vi "subFD_StructSel & CoefQuant.vi"() -> ()   [LabVIEW 2023]
uses:
  <vilib>/addons/Digital Filter Design/_Objects.llb/DFD Pole-Zero Plot.ctl
  <vilib>/addons/Digital Filter Design/_Objects.llb/DFD Filter Obj.ctl
  <vilib>/addons/Digital Filter Design/_Objects.llb/DFD Filter Coef.ctl
  <vilib>/addons/Digital Filter Design/_Objects.llb/DFD Filter Structure Type Selector.ctl
  <vilib>/addons/Digital Filter Design/_Objects.llb/dfd_Internal Quantization Settings.ctl
  <vilib>/addons/Digital Filter Design/_Objects.llb/dfd_Internal Quantization Srcs.ctl
  <vilib>/addons/Digital Filter Design/_Objects.llb/DFD Coef Norm Type.ctl
  <vilib>/addons/Digital Filter Design/_Objects.llb/DFD Phase Setting.ctl
  <vilib>/addons/Digital Filter Design/FXPModel.llb/DFD FXP Get Quantizer (All).vi
  <vilib>/addons/Digital Filter Design/FXPModel.llb/DFD FXP Quantize Coef (Easy).vi
  <vilib>/addons/Digital Filter Design/Analysis.llb/DFD Plot Freq Response (Linear-Spaced).vi
  <vilib>/addons/Digital Filter Design/NI_DigFilterLicensed.lvlib
panel:
  in  "Scale Type":u16(ring) items=["No Norm", "Time Domain 1-Norm", "Time Domain 2-Norm", "Time Domain Inf-Norm"]
  out "Status":string="Calculating........"
  in  "Scale Filter before Quantization":bool=TRUE
  in  "Coefficients a/k Word Length":i16=16 min=1 max=32 step=1
  in  "Coefficients b/v Word Length":i16=16 min=1 max=32 step=1
  out "Coefficients Report":string
  in  "Target Structure":u16(ring)=1 items=["FIR Direct Form"=1, "FIR Direct Form Transposed"=2, "FIR Symmetric"=3, "FIR Antisymmetric"=4, "IIR Direct Form I"=5, "IIR Direct Form I Transposed"=6, "IIR Direct Form II"=7, "IIR Direct Form II Transposed"=8, "IIR Cascaded Second-Order Sections Form I"=9, "IIR Cascaded Second-Order Sections Form I Transposed"=10, "IIR Cascaded Second-Order Sections Form II"=11, "IIR Cascaded Second-Order Sections Form II Transposed"=12, "Lattice Allpass (basic sections)"=13, "Lattice Allpass (one multiplier sections)"=14, "Lattice Allpass (normalized sections)"=15, "Lattice AR (basic sections)"=16, "Lattice AR (one multiplier sections)"=17, "Lattice AR (normalized sections)"=18, "Lattice MA (minimum phase)"=19, "Lattice MA (maximum phase)"=20, "Lattice ARMA (basic sections)"=21, "Lattice ARMA (one multiplier sections)"=22, "Lattice ARMA (normalized sections)"=23]
  out "Successful Design?":bool
  out "filter out":T1={"mSRate_Fs"=1.0, "mSRate_Version"="1.0", "mSRate_Comments"="", "mSRate_OrgCoef"={"type"=enum."Undefined", "gain"=1.0, "coef a (k)"=[], "coef b (v)"=[]}, "mSRate_CurCoef"={"type"=enum."Undefined", "gain"=1.0, "coef a (k)"=[], "coef b (v)"=[]}, "mSRate_Quantized?"=FALSE, "mSRate_QCoef"={"type"=enum."Undefined", "gain"=1.0, "coef a (k)"=[], "coef b (v)"=[]}, "mSRate_QSettings"=[], "mSRate_Order"=0, "mSRate_Scaling"={"mSRate_ScaleByPowerOf2?"=FALSE, "mSRate_ScaleType"=enum."No Norm"}} {"mSRate_QSettings"."source" items=["Coef a/k"=0, "Coef b/v"=7, "Input"=1, "Output"=2, "Multiplicand"=3, "Product"=4, "Sum"=5, "Delay"=6, "Gain"=8]}
  in  "filter in":T1={"mSRate_Fs"=1.0, "mSRate_Version"="1.0", "mSRate_Comments"="", "mSRate_OrgCoef"={"type"=enum."Undefined", "gain"=1.0, "coef a (k)"=[], "coef b (v)"=[]}, "mSRate_CurCoef"={"type"=enum."Undefined", "gain"=1.0, "coef a (k)"=[], "coef b (v)"=[]}, "mSRate_Quantized?"=FALSE, "mSRate_QCoef"={"type"=enum."Undefined", "gain"=1.0, "coef a (k)"=[], "coef b (v)"=[]}, "mSRate_QSettings"=[], "mSRate_Order"=0, "mSRate_Scaling"={"mSRate_ScaleByPowerOf2?"=FALSE, "mSRate_ScaleType"=enum."No Norm"}} {"mSRate_QSettings"."source" items=["Coef a/k"=0, "Coef b/v"=7, "Input"=1, "Output"=2, "Multiplicand"=3, "Product"=4, "Sum"=5, "Delay"=6, "Gain"=8]}
  in  "Graph Selector":u16(ring) items=["Magnitude", "Phase", "Group Delay", "Pole-Zero Plot", "Impulse Response"]
  in  "Unwrap?":bool=TRUE
  in  "Magnitude in dB?":bool=TRUE
  out "OK":bool
  in  "stop":bool
  out "Graph Tab":T7(tab)
  out "Magnitude Response":cluster{"f0":dbl, "df":dbl, "values":dbl[]}[](graph)
  out "Phase Response":cluster{"f0":dbl, "df":dbl, "values":dbl[]}[](graph)
  out "Group Delay":cluster{"f0":dbl, "df":dbl, "values":dbl[]}[](graph)
  out "Z-Plane":T8
  out "Coefficients":dbl[][](graph)
  # "Design Result"
  # "Target Structure"
  # "Coefficients Quantization Settings"
  # "Coefficients Report"
  # "Coefficients a/k\nWord Length"
  # "Coefficients b/v\nWord Length"
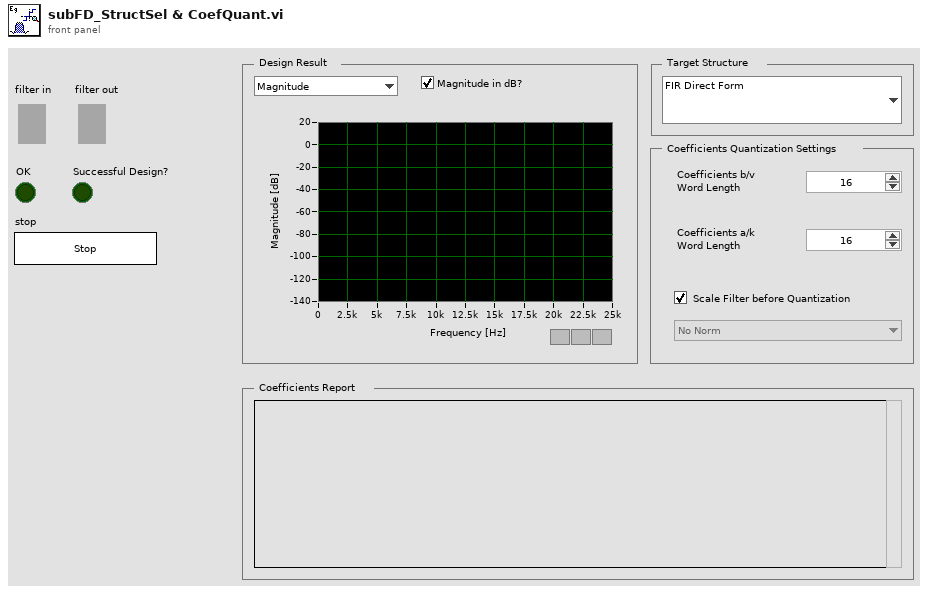
[diagram p1: front panel]
types:
  T1 = typedef "NI_DigFilterLicensed.lvlib/DFD Filter Obj.ctl" = cluster{"mSRate_Fs":dbl, "mSRate_Version":string, "mSRate_Comments":string, "mSRate_OrgCoef":T2, "mSRate_CurCoef":T2, "mSRate_Quantized?":bool, "mSRate_QCoef":T2, "mSRate_QSettings":T4[], "mSRate_Order":i32, "mSRate_Scaling":cluster{"mSRate_ScaleByPowerOf2?":bool, "mSRate_ScaleType":T6}}
  T2 = typedef "NI_DigFilterLicensed.lvlib/DFD Filter Coef.ctl" = cluster{"type":T3, "gain":dbl, "coef a (k)":dbl[], "coef b (v)":dbl[]}
  T3 = typedef "NI_DigFilterLicensed.lvlib/DFD Filter Structure Type Selector.ctl" = enum16{"Undefined", "FIR Direct Form", "FIR Direct Form Transposed", "FIR Symmetric", "FIR Antisymmetric", "IIR Direct Form I", "IIR Direct Form I Transposed", "IIR Direct Form II", "IIR Direct Form II Transposed", "IIR Cascaded Second Order Sections Form I", "IIR Cascaded Second Order Sections Form I Transposed", "IIR Cascaded Second Order Sections Form II", "IIR Cascaded Second Order Sections Form II Transposed", "Lattice Allpass (basic sections)", "Lattice Allpass (one multiplier sections)", "Lattice Allpass (normalized sections)", "Lattice AR (basic sections)", "Lattice AR (one multiplier sections)", "Lattice AR (normalized sections)", "Lattice MA (minimum phase)", "Lattice MA (maximum phase)", "Lattice ARMA (basic sections)", "Lattice ARMA (one multiplier sections)", "Lattice ARMA (normalized sections)"}
  T4 = typedef "NI_DigFilterLicensed.lvlib/dfd_Internal Quantization Settings.ctl" = cluster{"source":T5, "wl":i16, "iwl":i16, "overflow mode":enum16{"Saturation", "Wrap"}, "rounding mode":enum16{"Nearest", "Truncation"}, "signed?":bool}
  T5 = typedef "NI_DigFilterLicensed.lvlib/dfd_Internal Quantization Srcs.ctl" = u16
  T6 = typedef "NI_DigFilterLicensed.lvlib/DFD Coef Norm Type.ctl" = enum16{"No Norm", "Time Domain 1-Norm", "Time Domain 2-Norm", "Time Domain Inf-Norm"}
  T7 = enum32{"Magnitude", "Phase", "Group Delay", "Pole-Zero Plot", "Coefficients"}
  T8 = typedef "NI_DigFilterLicensed.lvlib/DFD Pole-Zero Plot.ctl" = cluster{dbl[], dbl[]}[]
  T9 = typedef "NI_DigFilterLicensed.lvlib/DFD Quantization Settings.ctl" = cluster{"source":T10, "wl":i16, "iwl":i16, "overflow mode":enum16{"Saturation", "Wrap"}, "rounding mode":enum16{"Nearest", "Truncation"}, "signed?":bool}
  T10 = typedef "NI_DigFilterLicensed.lvlib/DFD Quantization Sources.ctl" = u16
  T11 = typedef "NI_DigFilterLicensed.lvlib/DFD Phase Setting.ctl" = cluster{"unwrap? (F)":bool, "degree? (F)":bool}
  T12 = cluster{"t0":dbl, "dt":dbl, "amplitudes":dbl[]}[]
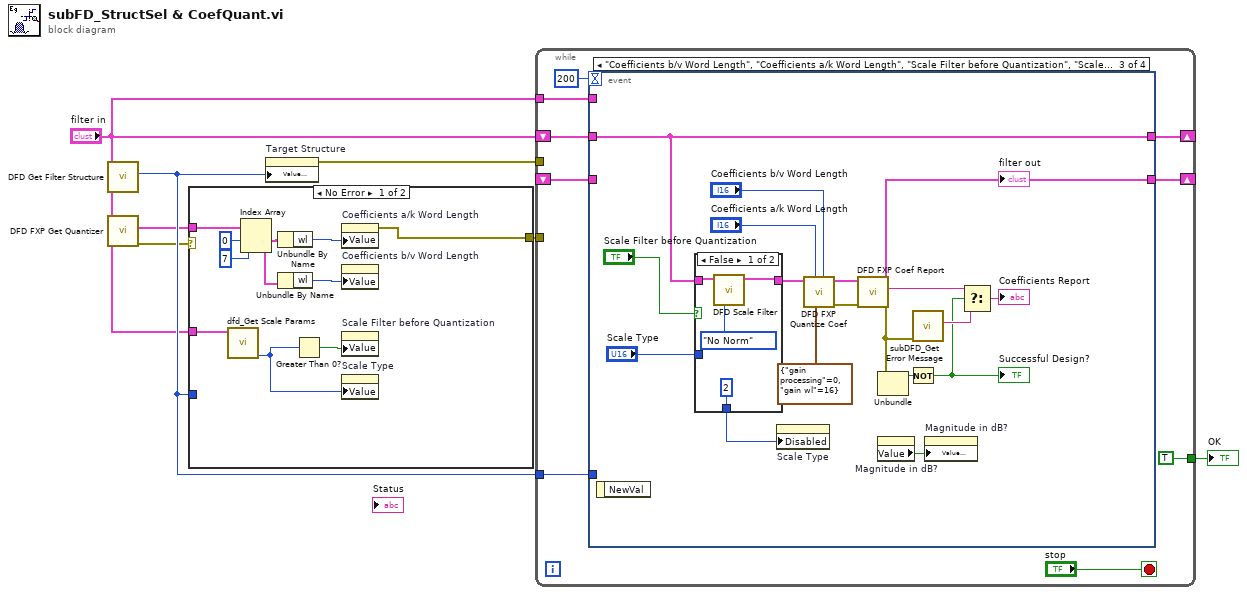
[diagram p0: block diagram]
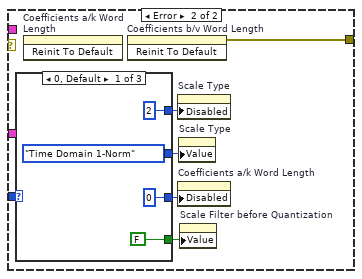
[diagram p2: hidden frame]
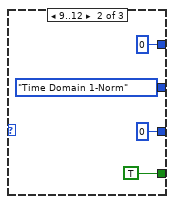
[diagram p3: hidden frame]
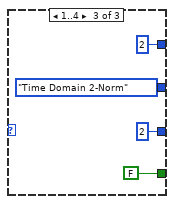
[diagram p4: hidden frame]
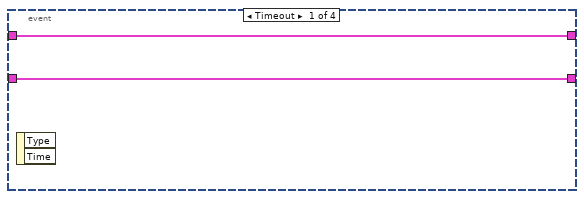
[diagram p5: hidden frame]
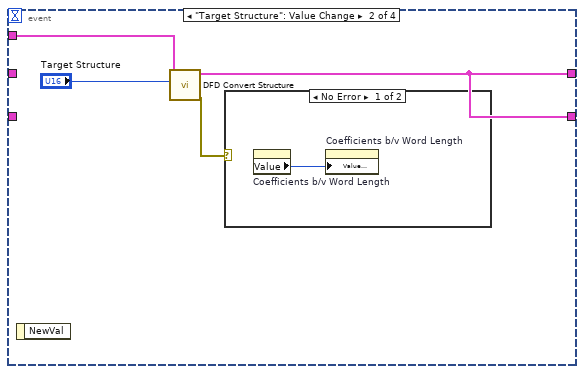
[diagram p6: hidden frame]
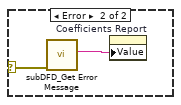
[diagram p7: hidden frame]
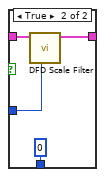
[diagram p8: hidden frame]
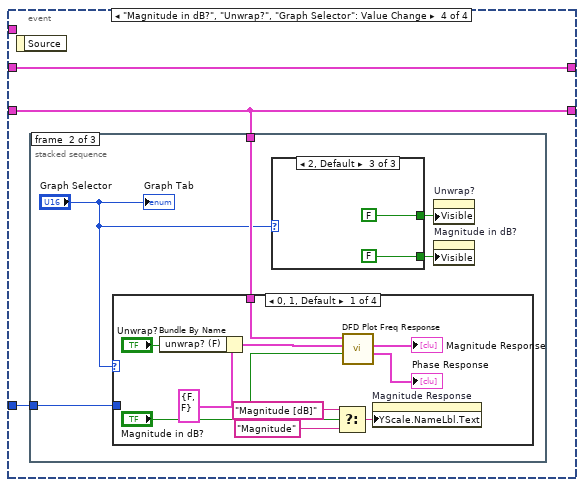
[diagram p9: hidden frame]
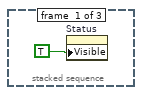
[diagram p10: hidden frame]
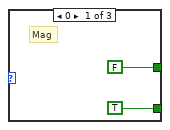
[diagram p11: hidden frame]
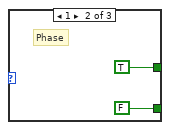
[diagram p12: hidden frame]
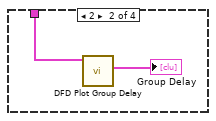
[diagram p13: hidden frame]
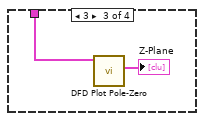
[diagram p14: hidden frame]
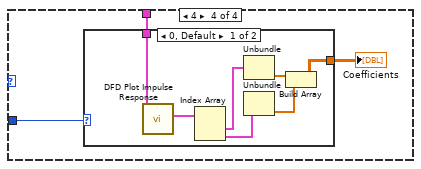
[diagram p15: hidden frame]
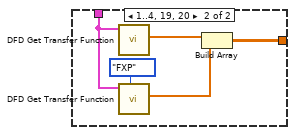
[diagram p16: hidden frame]
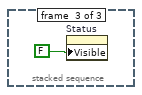
[diagram p17: hidden frame]
diagram:
  n1 = call <vilib>:"DFD Get Filter Structure.vi"("filter in"="filter in") -> ("structure"=w6:u16)  [unwired: 1 in, 9 out]
  n2 = call-poly <vilib>:"DFD FXP Get Quantizer.vi"("filter in"="filter in") -> ("error out"=w4:errorcluster, "quantizers"=w2:T9[])  [unwired: 1 in, 8 out]
  n3 = case shown="No Error" w4 {
    tunnel: w6 -> [_ w23]
    tunnel: [w11 w19] -> w3
    tunnel: w2 -> [w18 _]
    tunnel: "filter in" -> [w10 _]
    frame No Error {
      n4 = call <vilib>:"dfd_Get Scale Params.vi"("filter in"=w10) -> ("scale type"=w9:T6)  [unwired: 10 out]
      n5 = Index Array(array=w18, index #1=0 ("index"), index #2=7 ("index")) -> (element #1=w15:T9, element #2=w14:T9)
      n6 = Unbundle By Name(w15) -> ("wl"=w13:i16)
      n7 = Unbundle By Name(w14) -> ("wl"=w12:i16)
      n8 = Greater Than 0?(x=w9) -> (x > 0?=w8:bool)
      n9 = property on="Coefficients a/k Word Length" class="DigNum (strict)"("Value"=w13) -> (error out=w11:errorcluster)  [unwired: 2 in, 1 out]
      n10 = property on="Coefficients b/v Word Length" class="DigNum (strict)"("Value"=w12) -> ()  [unwired: 2 in, 2 out]
      n11 = property on="Scale Filter before Quantization" class="Bool (strict)"("Value"=w8) -> ()  [unwired: 2 in, 2 out]
      n12 = property on="Scale Type" class="Ring (strict)"("Value"=w9) -> ()  [unwired: 2 in, 2 out]
    }
    frame Error {
      n13 = case shown="0, Default" w23 {
        tunnel: [u8 0 ("Disabled") u8 0 ("Disabled") u8 2 ("Disabled")] -> w24
        tunnel: [DFD_Coef_Norm_Type."Time Domain 1-Norm" ("scale type") DFD_Coef_Norm_Type."Time Domain 1-Norm" ("scale type") DFD_Coef_Norm_Type."Time Domain 2-Norm" ("scale type")] -> w22
        tunnel: [FALSE TRUE FALSE] -> w21
        tunnel: [u8 2 ("Disabled") u8 0 ("Disabled") u8 2 ("Disabled")] -> w20
        frame 0, Default {
        }
        frame 9..12 {
        }
        frame 1..4 {
        }
      }
      n14 = invoke on="Coefficients a/k Word Length" class="DigNum (strict)" method="Reinit To Default"() -> ()  [unwired: 3 in, 3 out]
      n15 = invoke on="Coefficients b/v Word Length" class="DigNum (strict)" method="Reinit To Default"() -> (error out=w19:errorcluster)  [unwired: 3 in, 2 out]
      n16 = property on="Scale Type" class="Ring (strict)"("Disabled"=w20) -> ()  [unwired: 2 in, 2 out]
      n17 = property on="Coefficients a/k Word Length" class="DigNum (strict)"("Disabled"=w24) -> ()  [unwired: 2 in, 2 out]
      n18 = property on="Scale Type" class="Ring (strict)"("Value"=w22) -> ()  [unwired: 2 in, 2 out]
      n19 = property on="Scale Filter before Quantization" class="Bool (strict)"("Value"=w21) -> ()  [unwired: 2 in, 2 out]
    }
  }
  n20 = property on="Target Structure" class="Ring (strict)"("Value (Signaling)"=w6) -> (error out=w5:errorcluster)  [unwired: 2 in, 1 out]
  n21 = while {
    tunnel: [TRUE] -> w7
    shift-right: [w41] -> _
    shift-left: "filter in" -> [w42]
    tunnel: w6 -> [w40]
    tunnel: "filter in" -> [w39]
    tunnel: w5 -> [_]
    shift-right: [w38] -> _
    shift-left: _ -> [w37]
    tunnel: w3 -> [_]
    stop <- "stop" stop-if-true
    n22 = event shown="[2] \"Coefficients b/v Word Length\", \"Coefficients a/k Word Length\", \"Scale Filter before Quantization\", \"Scale Type\": Value Change" {
      selector: _ -> [_ _ _ _]
      dyn-events: _ -> [_ _ _ _]
      timeout: 200 -> [_ _ _ _]
      tunnel: w42 -> [w47 _ w71 w82]
      tunnel: [w47 w48 w71 w82] -> w41
      tunnel: w40 -> [_ _ _ w83]
      tunnel: w39 -> [_ w50 _ _]
      tunnel: [w46 w48 w72 w81] -> w38
      tunnel: w37 -> [w46 _ _ w81]
      event Timeout {
        n23 = event-data() -> ()  [unwired: 3 out]
      }
      event "Target Structure": Value Change {
        n24 = event-data() -> ()  [unwired: 2 out]
        n25 = call <vilib>:"DFD Convert Structure.vi"("target structure"="Target Structure", "filter in"=w50) -> ("error out"=w49:errorcluster, "filter out"=w48:T1)  [unwired: 1 in, 7 out]
        n26 = case shown="No Error" w49 {
          selector: w49 -> [_ w54]
          frame No Error {
            n27 = property on="Coefficients b/v Word Length" class="DigNum (strict)"() -> ("Value"=w52:i16)  [unwired: 2 in, 2 out]
            n28 = property on="Coefficients b/v Word Length" class="DigNum (strict)"("Value (Signaling)"=w52) -> ()  [unwired: 2 in, 2 out]
          }
          frame Error {
            n29 = call <vilib>:"subDFD_Get Error Message.vi"("error in (no error)"=w54) -> ("Error Message"=w53:string)  [unwired: 10 out]
            n30 = property on="Coefficients Report" class="Str"("Value"=w53) -> ()  [unwired: 2 in, 2 out]
          }
        }
      }
      event "Coefficients b/v Word Length", "Coefficients a/k Word Length", "Scale Filter before Quantization", "Scale Type": Value Change {
        n31 = event-data() -> ()  [unwired: 2 out]
        n32 = case shown="False" "Scale Filter before Quantization" {
          tunnel: w71 -> [w75 w80]
          tunnel: [w74 w79] -> w58
          tunnel: "Scale Type" -> [_ w78]
          tunnel: [u8 2 ("Disabled") u8 0 ("Disabled")] -> w55
          frame False {
            n33 = call <vilib>:"DFD Scale Filter.vi"("scale type"=DFD_Coef_Norm_Type."No Norm", "filter in"=w75) -> ("filter out"=w74:T1)  [unwired: 1 in, 8 out]
          }
          frame True {
            n34 = call <vilib>:"DFD Scale Filter.vi"("scale type"=w78, "filter in"=w80) -> ("filter out"=w79:T1)  [unwired: 1 in, 8 out]
          }
        }
        n35 = property on="Scale Type" class="Ring (strict)"("Disabled"=w55) -> ()  [unwired: 2 in, 2 out]
        n36 = call-poly <vilib>:"DFD FXP Quantize Coef.vi"("coefficients b/v word length"="Coefficients b/v Word Length", "gain settings"=cluster{"gain processing":u16, "gain wl":i16} {"gain processing"=0, "gain wl"=16}, "coefficients a/k word length"="Coefficients a/k Word Length", "filter in"=w58) -> ("error out"=w68:errorcluster, "filter out"=w69:T1)  [unwired: 1 in, 5 out]
        n37 = call <vilib>:"DFD FXP Coef Report.vi"("error in (no error)"=w68, "filter in"=w69) -> ("error out"=w66:errorcluster, "coefficients report"=w65:string, "filter out"=w72:T1)  [unwired: 7 out]
        "filter out" <- w72
        n38 = Unbundle(w66) -> ("status"=w67:bool)  [unwired: 2 out]
        n39 = property on="Magnitude in dB?" class="Bool (strict)"() -> ("Value"=w70:bool)  [unwired: 2 in, 2 out]
        n40 = Not(x=w67) -> (.not. x?=w59:bool)
        "Successful Design?" <- w59
        n41 = call <vilib>:"subDFD_Get Error Message.vi"("error in (no error)"=w66) -> ("Error Message"=w64:string)  [unwired: 10 out]
        n42 = property on="Magnitude in dB?" class="Bool (strict)"("Value (Signaling)"=w70) -> ()  [unwired: 2 in, 2 out]
        n43 = Select(t=w65, s=w59, f=w64) -> (s? t:f=→"Coefficients Report":string)
      }
      event "Magnitude in dB?", "Unwrap?", "Graph Selector": Value Change {
        n44 = event-data() -> ()  [unwired: 2 out]
        n45 = stacked-sequence {
          tunnel: w83 -> [_ w89 _]
          tunnel: w81 -> [_ w88 _]
          frame #0 {
            n46 = property on="Status" class="Str"("Visible"=TRUE) -> ()  [unwired: 2 in, 2 out]
          }
          frame #1 {
            n47 = case shown="0, 1, Default" "Graph Selector" {
              tunnel: w89 -> [_ _ _ w111]
              tunnel: w88 -> [w100 w106 w108 w110]
              frame 0, 1, Default {
                n48 = Bundle By Name(cluster=T11 {"unwrap? (F)"=FALSE, "degree? (F)"=FALSE} ("phase view"), "unwrap? (F)"="Unwrap?") -> (w101:T11)
                n49 = Select(t="Magnitude [dB]", s="Magnitude in dB?", f="Magnitude") -> (s? t:f=w96:string)
                n50 = call-poly <vilib>:"DFD Plot Freq Response.vi"("dB on? (T)"="Magnitude in dB?", "phase view"=w101, "filter in"=w100) -> ("phase response"=→"Phase Response":cluster{"f0":dbl, "df":dbl, "values":dbl[]}[], "magnitude response"=→"Magnitude Response":cluster{"f0":dbl, "df":dbl, "values":dbl[]}[])  [unwired: 5 in, 2 out]
                n51 = property on="Magnitude Response" class="WFGraph (strict)"("YScale.NameLbl.Text"=w96) -> ()  [unwired: 2 in, 2 out]
              }
              frame 2 {
                n52 = call <vilib>:"DFD Plot Group Delay.vi"("filter in"=w106) -> ("group delay"=→"Group Delay":cluster{"f0":dbl, "df":dbl, "values":dbl[]}[])  [unwired: 3 in, 7 out]
              }
              frame 3 {
                n53 = call <vilib>:"DFD Plot Pole-Zero.vi"("filter in"=w108) -> ("Z-Plane"=→"Z-Plane":T8)  [unwired: 2 in, 8 out]
              }
              frame 4 {
                n54 = case shown="0, Default" w111 {
                  tunnel: w110 -> [w119 w120]
                  tunnel: [w113 w121] -> w112
                  frame 0, Default {
                    n55 = call <vilib>:"DFD Plot Impulse Response.vi"("filter in"=w119) -> ("impulse response"=w118:T12)  [unwired: 3 in, 7 out]
                    n56 = Index Array(array=w118) -> (element #1=w117:cluster{"t0":dbl, "dt":dbl, "amplitudes":dbl[]}, element #2=w116:cluster{"t0":dbl, "dt":dbl, "amplitudes":dbl[]})  [unwired: 2 in]
                    n57 = Unbundle(w117) -> ("amplitudes"=w115:dbl[])  [unwired: 2 out]
                    n58 = Unbundle(w116) -> ("amplitudes"=w114:dbl[])  [unwired: 2 out]
                    n59 = Build Array(w115, w114) -> (w113:dbl[][])
                  }
                  frame 1..4, 19, 20 {
                    n60 = call <vilib>:"DFD Get Transfer Function.vi"("filter in"=w120) -> ("numerator"=w123:dbl[])  [unwired: 1 in, 9 out]
                    n61 = call <vilib>:"DFD Get Transfer Function.vi"("type (FLP)"=enum16{"FLP", "FXP"}."FXP", "filter in"=w120) -> ("numerator"=w122:dbl[])  [unwired: 1 in, 8 out]
                    n62 = Build Array(w123, w122) -> (w121:dbl[][])
                  }
                }
                "Coefficients" <- w112
              }
            }
            n63 = case shown="2, Default" "Graph Selector" {
              tunnel: [FALSE TRUE FALSE] -> w87
              tunnel: [TRUE FALSE FALSE] -> w86
              frame 0 {
                # "Mag"
              }
              frame 1 {
                # "Phase"
              }
              frame 2, Default {
              }
            }
            n64 = property on="Unwrap?" class="Bool (strict)"("Visible"=w87) -> ()  [unwired: 2 in, 2 out]
            n65 = property on="Magnitude in dB?" class="Bool (strict)"("Visible"=w86) -> ()  [unwired: 2 in, 2 out]
            "Graph Tab" <- "Graph Selector"
          }
          frame #2 {
            n66 = property on="Status" class="Str"("Visible"=FALSE) -> ()  [unwired: 2 in, 2 out]
          }
        }
      }
    }
  }
  "OK" <- w7
